vi "WPI_GyroOpen.vi"   [LabVIEW 2017]
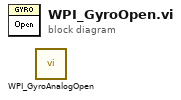
[diagram p0: block diagram]
diagram:
  n1 = call <vilib>:"WPI_GyroAnalogOpen.vi"() -> ()  [unwired: 9 in, 3 out]
